vi "Abort Recipe.vi"(8 "error in (no error)":errorcluster, 11 "Recipe Controller in":refnum<class "Recipe Controller.lvclass">) -> (0 "error out":errorcluster, 3 "Recipe Controller out":refnum<class "Recipe Controller.lvclass">)   [LabVIEW 2022 SP3, in "Recipe Controller.lvclass"]
uses:
  Recipe Controller.lvclass
  Recipe Controller.lvclass/Recipe Controller.ctl
  XY Stage/Process Actor/Process Framework/Process State Data/Process State Data.lvclass/Process State Data.ctl
  XY Stage/Process Actor/Process Framework/Interlock Q Class/Interlock Q Class.lvclass/Interlock Q Class.ctl
  <vilib>/ActorFramework/Message Enqueuer/Message Enqueuer.lvclass/Message Enqueuer.ctl
  XY Stage/Process Actor/Process Framework/Process State Data/Accessor/Write Abort.vi
  <vilib>/ActorFramework/Message Enqueuer/Enqueue.vi
  Recipe Process/Recipe Process Messages/Abort Recipe Msg/Abort Recipe Msg.lvclass
  C:/Program Files/National Instruments/LabVIEW 2022/vi.lib/ActorFramework/Message/Message.lvclass
  <vilib>/ActorFramework/Message Priority Queue/Priority Enqueue.vi
  <vilib>/ActorFramework/Message Enqueuer/Message Enqueuer.lvclass
  XY Stage/Process Actor/Process Framework/Interlock Q Class/Interlock Q Class.lvclass
  XY Stage/Process Actor/Process Framework/Process State Data/Process State Data.lvclass
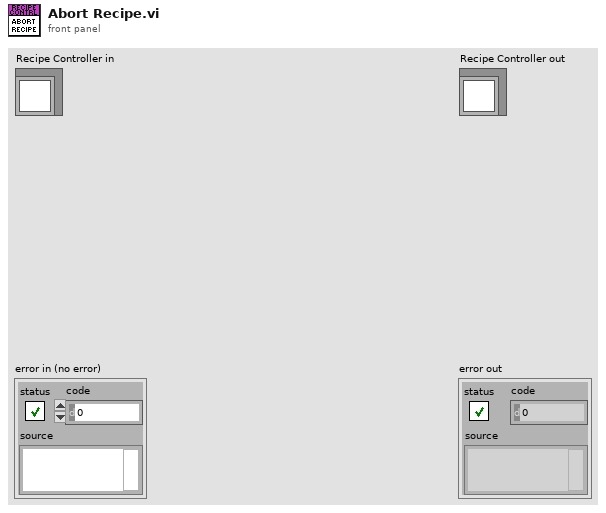
[diagram p1: front panel]
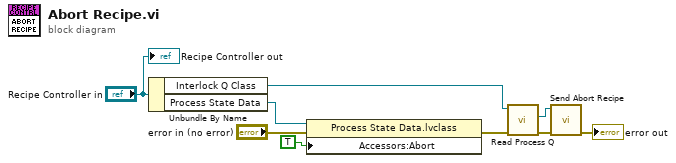
[diagram p0: block diagram]
diagram:
  n1 = Unbundle By Name("Recipe Controller in") -> ("Interlock Q Class"=w8:refnum<class "Interlock Q Class.lvclass">, "Process State Data"=w6:refnum<data-value>)
  n2 = property class="Process State Data.lvclass"(reference=w6, error in="error in (no error)", "Accessors:Abort"=TRUE ("Abort")) -> (error out=w3:errorcluster)  [unwired: 1 out]
  n3 = call "Read Process Q.vi"("error in (no error)"=w3, "Interlock Q Class in"=w8) -> ("error out"=w2:errorcluster, "Actor Framework:Message Enqueuer"=w7:refnum<class "Message Enqueuer.lvclass">)  [unwired: 7 in, 1 out]
  n4 = call "Send Abort Recipe.vi"("error in (no error)"=w2, "Message Enqueuer"=w7) -> ("error out"=→"error out":errorcluster)  [unwired: 8 in, 1 out]
  "Recipe Controller out" <- "Recipe Controller in"
